vi "Configure Range.vi"(0 "VISA resource name":refnum<visa-resource-name>, 5 "Range Index (0)":u32, 11 "error in (no error)":errorcluster) -> (4 "VISA resource name out":refnum<visa-resource-name>, 15 "error out":errorcluster)   [LabVIEW 2020, in "NH Research Regenerative Test Series.lvlib"]
doc: "Sets the active range using a zero-based index. Use <B>Query Capabilities (Range)</B> to determine the maximum number of ranges."
uses:
  NH Research Regenerative Test Series.lvlib
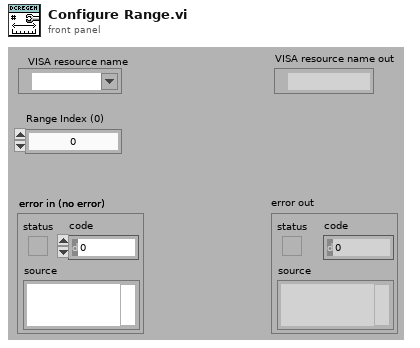
[diagram p1: front panel]
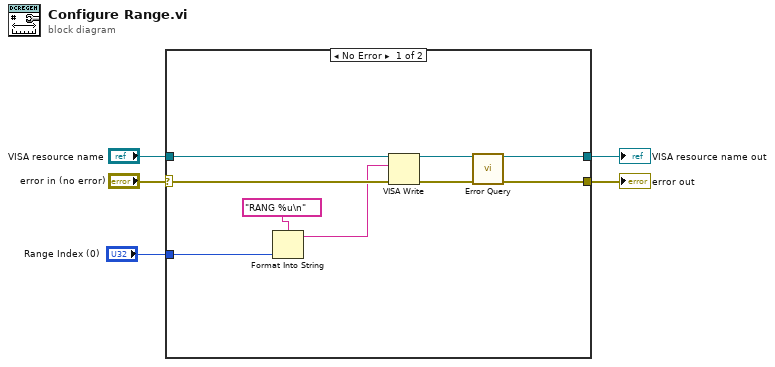
[diagram p0: block diagram]
diagram:
  n1 = case shown="No Error" "error in (no error)" {
    selector: "error in (no error)" -> [w9 w16]
    tunnel: "VISA resource name" -> [w14 w15]
    tunnel: [w13 w15] -> w4
    tunnel: [w12 w16] -> w3
    tunnel: "Range Index (0)" -> [w6 _]
    frame No Error {
      n2 = Format Into String(format string="RANG %u\n", w6) -> (resulting string=w7:string)  [unwired: 2 in, 1 out]
      n3 = VISA Write(VISA resource name=w14, write buffer=w7, error in (no error)=w9) -> (VISA resource name out=w11:refnum<visa-resource-name>, error out=w10:errorcluster)  [unwired: 1 out]
      n4 = call "Error Query.vi"("VISA resource name"=w11, "error in (no error)"=w10) -> ("VISA resource name out"=w13:refnum<visa-resource-name>, "error out"=w12:errorcluster)  [unwired: 10 in, 2 out]
    }
    frame Error {
    }
  }
  "error out" <- w3
  "VISA resource name out" <- w4
